vi "SpectrumAnn SCPI commands.vi"(11 "Path":path) -> (0 "error out":errorcluster, 2 "result string":string="3-19-2018", 3 "VISA Refnum out":refnum<visa-resource-name>)   [LabVIEW 2017]
uses:
  <vilib>/regexp/Match Regular Expression.xnode
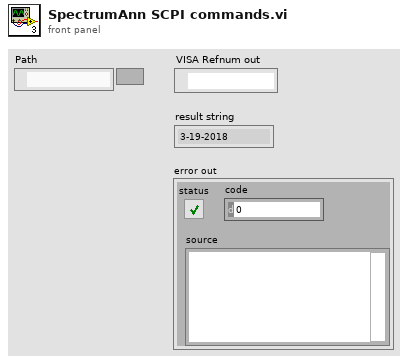
[diagram p1: front panel]
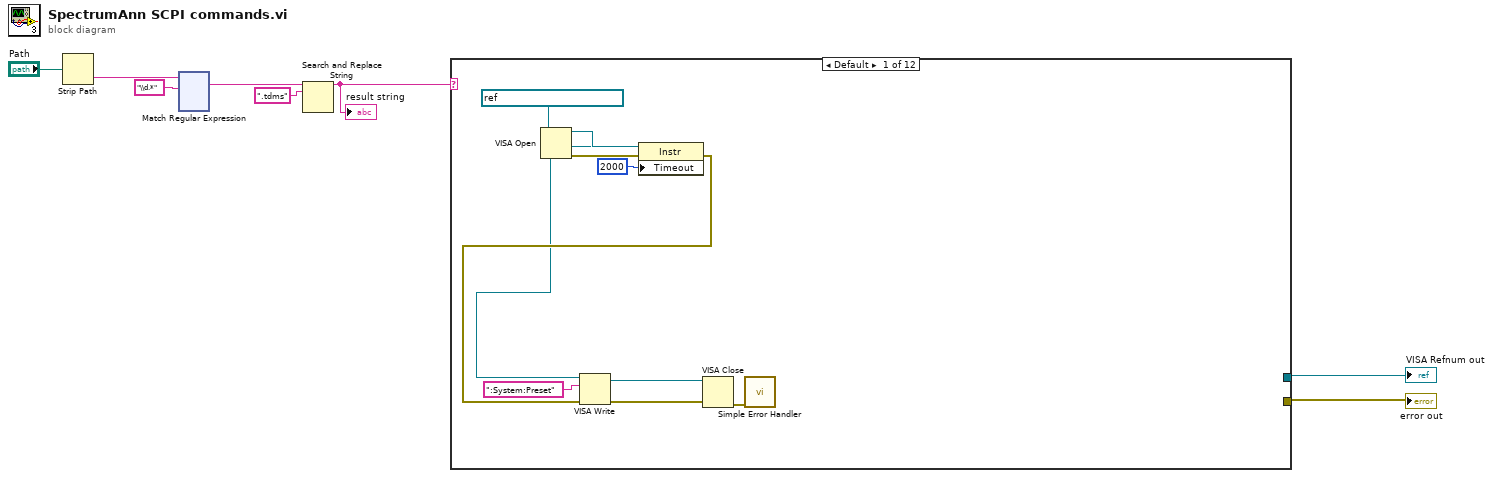
[diagram p0: block diagram]
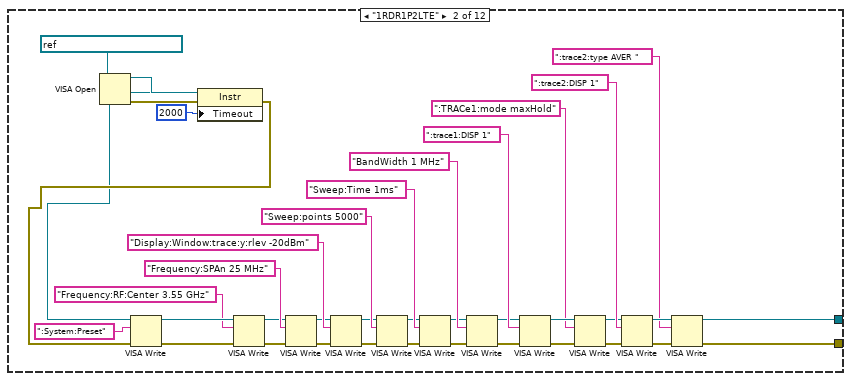
[diagram p2: hidden frame]
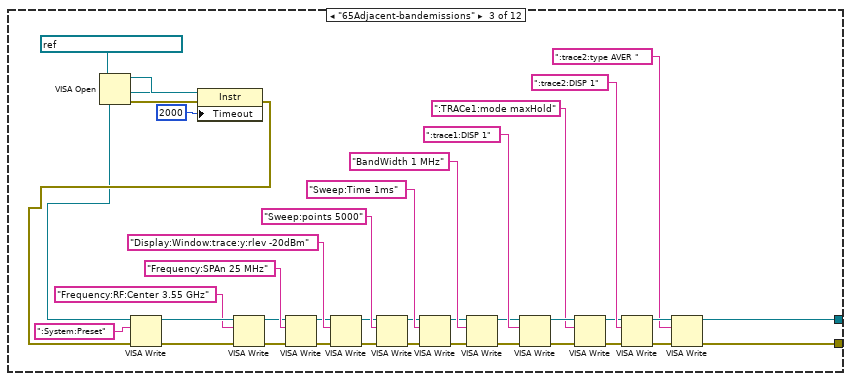
[diagram p3: hidden frame]
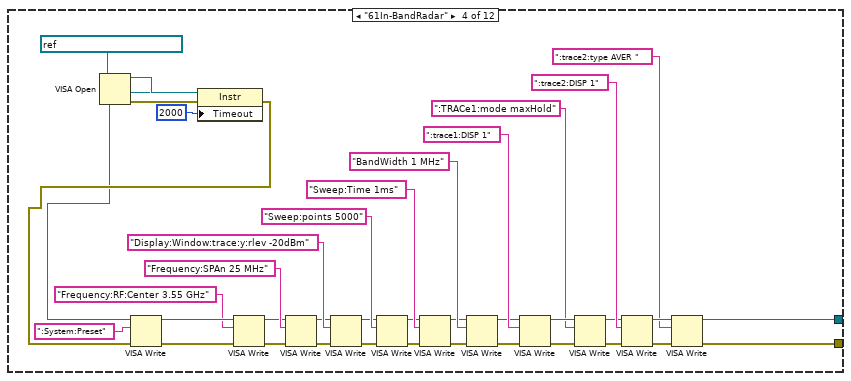
[diagram p4: hidden frame]
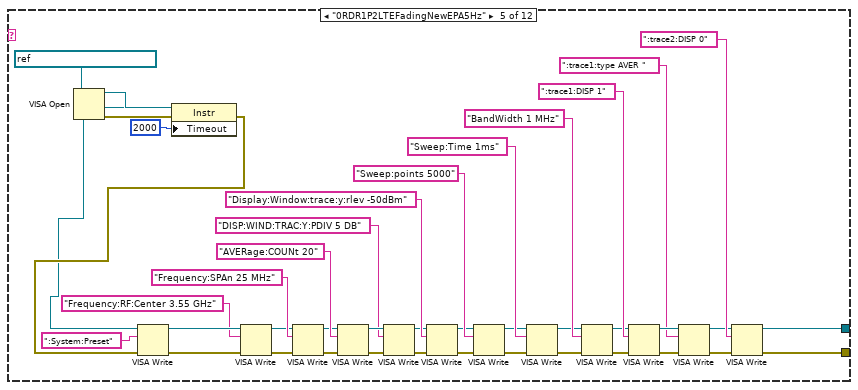
[diagram p5: hidden frame]
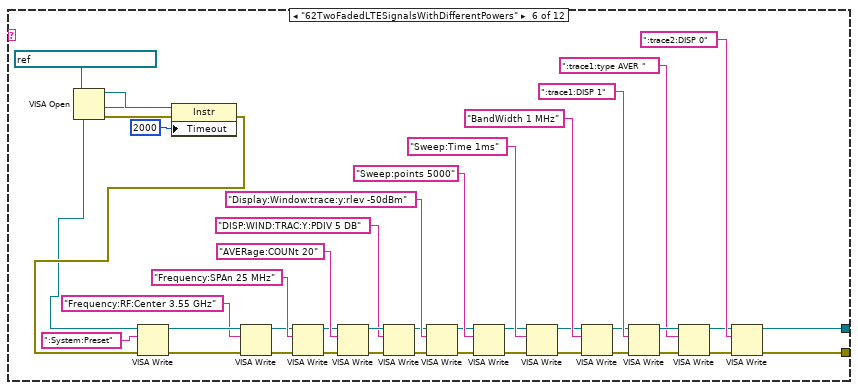
[diagram p6: hidden frame]
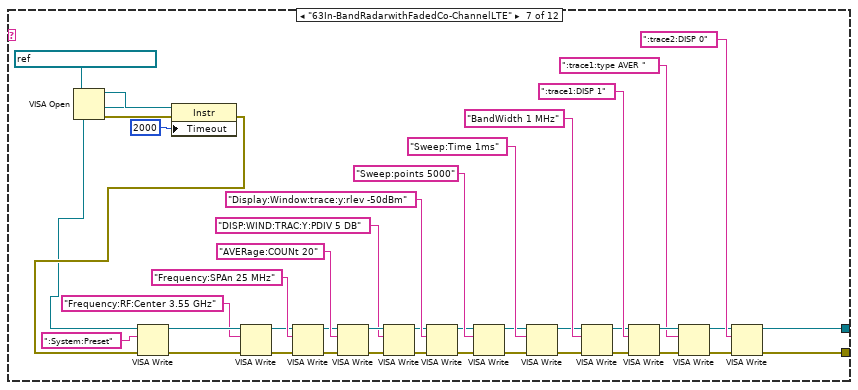
[diagram p7: hidden frame]
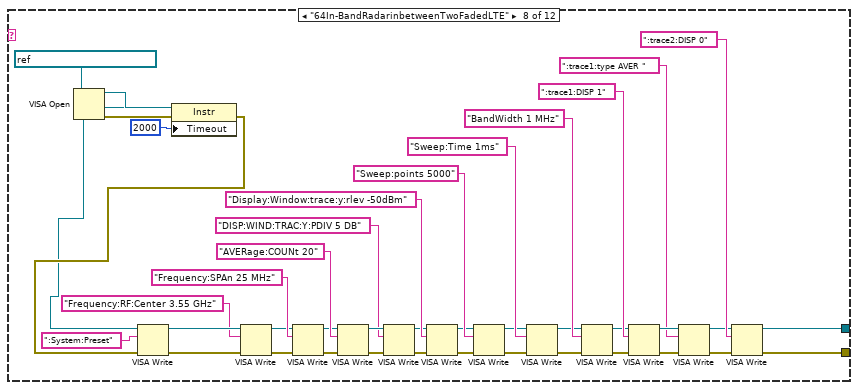
[diagram p8: hidden frame]
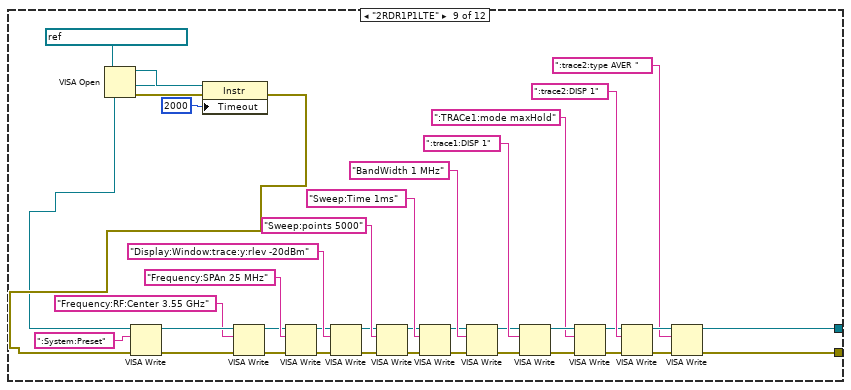
[diagram p9: hidden frame]
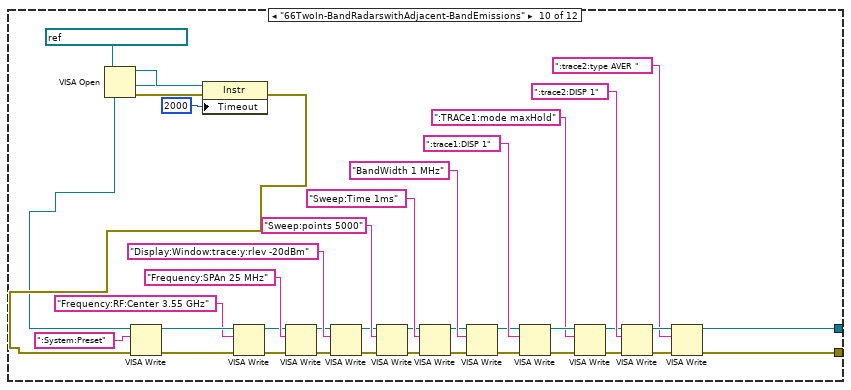
[diagram p10: hidden frame]
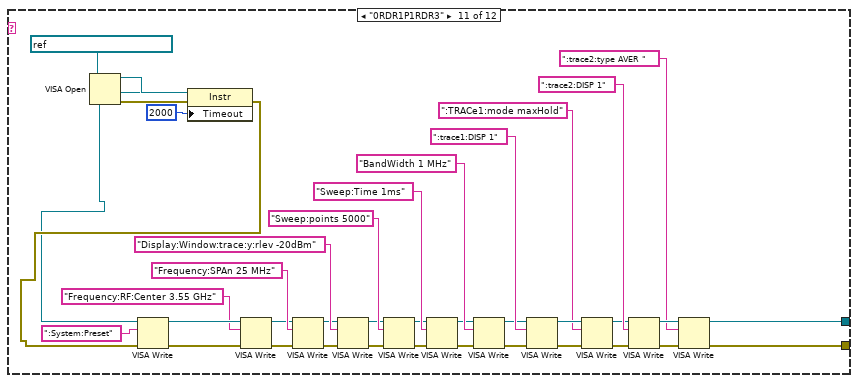
[diagram p11: hidden frame]
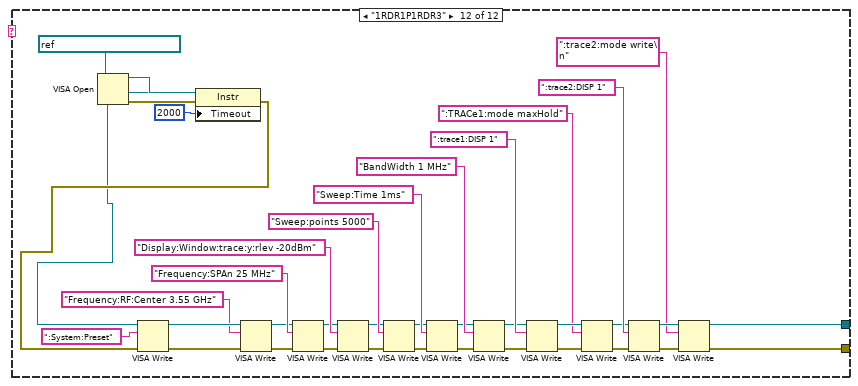
[diagram p12: hidden frame]
diagram:
  n1 = Strip Path(path="Path") -> (name=w5:string)  [unwired: 1 out]
  n2 = xnode "Match Regular Expression"("input string"=w5, "regular expression"="\\d.*") -> ("whole match"=w1:string)  [unwired: 4 in, 4 out]
  n3 = Search and Replace String(input string=w1, search string=".tdms") -> (result string=w6:string)  [unwired: 6 in, 3 out]
  "result string" <- w6
  n4 = case shown="Default" w6 {
    tunnel: [_ w25 w64 w103 w143 w185 w227 w269 w311 w350 w389 w428] -> w7
    tunnel: [_ w26 w65 w104 w142 w184 w226 w268 w310 w349 w388 w427] -> w8
    frame Default {
      n5 = VISA Open(VISA resource name=refnum<visa-resource-name> "SpecAnn-9010A-20100") -> (VISA resource name=w16:refnum<visa-resource-name>, error out=w15:errorcluster)  [unwired: 4 in]
      n6 = property class="Instr"(reference=w16, error in=w15, "Timeout"=u32 2000 ("General Settings:Timeout Value")) -> (reference out=w12:refnum<visa-resource-name>, error out=w13:errorcluster)
      n7 = VISA Write(VISA resource name=w12, write buffer=":System:Preset", error in (no error)=w13) -> (VISA resource name out=w10:refnum<visa-resource-name>, error out=w9:errorcluster)  [unwired: 1 out]
      n8 = VISA Close(VISA resource name=w10, error in (no error)=w9) -> (error out=w11:errorcluster)
      n9 = call <vilib>:"Simple Error Handler.vi"("error in (no error)"=w11) -> ()  [unwired: 4 in, 5 out]
    }
    frame "1RDR1P2LTE" {
      n10 = VISA Open(VISA resource name=refnum<visa-resource-name> "SpecAnn-9010A-20100") -> (VISA resource name=w23:refnum<visa-resource-name>, error out=w22:errorcluster)  [unwired: 4 in]
      n11 = property class="Instr"(reference=w23, error in=w22, "Timeout"=u32 2000 ("General Settings:Timeout Value")) -> (reference out=w19:refnum<visa-resource-name>, error out=w20:errorcluster)
      n12 = VISA Write(VISA resource name=w19, write buffer=":System:Preset", error in (no error)=w20) -> (VISA resource name out=w47:refnum<visa-resource-name>, error out=w46:errorcluster)  [unwired: 1 out]
      n13 = VISA Write(VISA resource name=w47, write buffer="Frequency:RF:Center 3.55 GHz", error in (no error)=w46) -> (VISA resource name out=w39:refnum<visa-resource-name>, error out=w30:errorcluster)  [unwired: 1 out]
      n14 = VISA Write(VISA resource name=w39, write buffer="Frequency:SPAn 25 MHz", error in (no error)=w30) -> (VISA resource name out=w38:refnum<visa-resource-name>, error out=w31:errorcluster)  [unwired: 1 out]
      n15 = VISA Write(VISA resource name=w38, write buffer="Display:Window:trace:y:rlev -20dBm", error in (no error)=w31) -> (VISA resource name out=w37:refnum<visa-resource-name>, error out=w32:errorcluster)  [unwired: 1 out]
      n16 = VISA Write(VISA resource name=w37, write buffer="Sweep:points 5000", error in (no error)=w32) -> (VISA resource name out=w36:refnum<visa-resource-name>, error out=w33:errorcluster)  [unwired: 1 out]
      n17 = VISA Write(VISA resource name=w36, write buffer="Sweep:Time 1ms", error in (no error)=w33) -> (VISA resource name out=w35:refnum<visa-resource-name>, error out=w34:errorcluster)  [unwired: 1 out]
      n18 = VISA Write(VISA resource name=w35, write buffer="BandWidth 1 MHz", error in (no error)=w34) -> (VISA resource name out=w28:refnum<visa-resource-name>, error out=w29:errorcluster)  [unwired: 1 out]
      n19 = VISA Write(VISA resource name=w28, write buffer=":trace1:DISP 1", error in (no error)=w29) -> (VISA resource name out=w53:refnum<visa-resource-name>, error out=w52:errorcluster)  [unwired: 1 out]
      n20 = VISA Write(VISA resource name=w53, write buffer=":TRACe1:mode maxHold", error in (no error)=w52) -> (VISA resource name out=w50:refnum<visa-resource-name>, error out=w49:errorcluster)  [unwired: 1 out]
      n21 = VISA Write(VISA resource name=w50, write buffer=":trace2:DISP 1", error in (no error)=w49) -> (VISA resource name out=w56:refnum<visa-resource-name>, error out=w57:errorcluster)  [unwired: 1 out]
      n22 = VISA Write(VISA resource name=w56, write buffer=":trace2:type AVER ", error in (no error)=w57) -> (VISA resource name out=w25:refnum<visa-resource-name>, error out=w26:errorcluster)  [unwired: 1 out]
    }
    frame "65Adjacent-bandemissions" {
      n23 = VISA Open(VISA resource name=refnum<visa-resource-name> "SpecAnn-9010A-20100") -> (VISA resource name=w62:refnum<visa-resource-name>, error out=w61:errorcluster)  [unwired: 4 in]
      n24 = property class="Instr"(reference=w62, error in=w61, "Timeout"=u32 2000 ("General Settings:Timeout Value")) -> (reference out=w58:refnum<visa-resource-name>, error out=w59:errorcluster)
      n25 = VISA Write(VISA resource name=w58, write buffer=":System:Preset", error in (no error)=w59) -> (VISA resource name out=w86:refnum<visa-resource-name>, error out=w85:errorcluster)  [unwired: 1 out]
      n26 = VISA Write(VISA resource name=w86, write buffer="Frequency:RF:Center 3.55 GHz", error in (no error)=w85) -> (VISA resource name out=w78:refnum<visa-resource-name>, error out=w69:errorcluster)  [unwired: 1 out]
      n27 = VISA Write(VISA resource name=w78, write buffer="Frequency:SPAn 25 MHz", error in (no error)=w69) -> (VISA resource name out=w77:refnum<visa-resource-name>, error out=w70:errorcluster)  [unwired: 1 out]
      n28 = VISA Write(VISA resource name=w77, write buffer="Display:Window:trace:y:rlev -20dBm", error in (no error)=w70) -> (VISA resource name out=w76:refnum<visa-resource-name>, error out=w71:errorcluster)  [unwired: 1 out]
      n29 = VISA Write(VISA resource name=w76, write buffer="Sweep:points 5000", error in (no error)=w71) -> (VISA resource name out=w75:refnum<visa-resource-name>, error out=w72:errorcluster)  [unwired: 1 out]
      n30 = VISA Write(VISA resource name=w75, write buffer="Sweep:Time 1ms", error in (no error)=w72) -> (VISA resource name out=w74:refnum<visa-resource-name>, error out=w73:errorcluster)  [unwired: 1 out]
      n31 = VISA Write(VISA resource name=w74, write buffer="BandWidth 1 MHz", error in (no error)=w73) -> (VISA resource name out=w67:refnum<visa-resource-name>, error out=w68:errorcluster)  [unwired: 1 out]
      n32 = VISA Write(VISA resource name=w67, write buffer=":trace1:DISP 1", error in (no error)=w68) -> (VISA resource name out=w92:refnum<visa-resource-name>, error out=w91:errorcluster)  [unwired: 1 out]
      n33 = VISA Write(VISA resource name=w92, write buffer=":TRACe1:mode maxHold", error in (no error)=w91) -> (VISA resource name out=w89:refnum<visa-resource-name>, error out=w88:errorcluster)  [unwired: 1 out]
      n34 = VISA Write(VISA resource name=w89, write buffer=":trace2:DISP 1", error in (no error)=w88) -> (VISA resource name out=w95:refnum<visa-resource-name>, error out=w96:errorcluster)  [unwired: 1 out]
      n35 = VISA Write(VISA resource name=w95, write buffer=":trace2:type AVER ", error in (no error)=w96) -> (VISA resource name out=w64:refnum<visa-resource-name>, error out=w65:errorcluster)  [unwired: 1 out]
    }
    frame "61In-BandRadar" {
      n36 = VISA Open(VISA resource name=refnum<visa-resource-name> "SpecAnn-9010A-20100") -> (VISA resource name=w101:refnum<visa-resource-name>, error out=w100:errorcluster)  [unwired: 4 in]
      n37 = property class="Instr"(reference=w101, error in=w100, "Timeout"=u32 2000 ("General Settings:Timeout Value")) -> (reference out=w97:refnum<visa-resource-name>, error out=w98:errorcluster)
      n38 = VISA Write(VISA resource name=w97, write buffer=":System:Preset", error in (no error)=w98) -> (VISA resource name out=w125:refnum<visa-resource-name>, error out=w124:errorcluster)  [unwired: 1 out]
      n39 = VISA Write(VISA resource name=w125, write buffer="Frequency:RF:Center 3.55 GHz", error in (no error)=w124) -> (VISA resource name out=w117:refnum<visa-resource-name>, error out=w108:errorcluster)  [unwired: 1 out]
      n40 = VISA Write(VISA resource name=w117, write buffer="Frequency:SPAn 25 MHz", error in (no error)=w108) -> (VISA resource name out=w116:refnum<visa-resource-name>, error out=w109:errorcluster)  [unwired: 1 out]
      n41 = VISA Write(VISA resource name=w116, write buffer="Display:Window:trace:y:rlev -20dBm", error in (no error)=w109) -> (VISA resource name out=w115:refnum<visa-resource-name>, error out=w110:errorcluster)  [unwired: 1 out]
      n42 = VISA Write(VISA resource name=w115, write buffer="Sweep:points 5000", error in (no error)=w110) -> (VISA resource name out=w114:refnum<visa-resource-name>, error out=w111:errorcluster)  [unwired: 1 out]
      n43 = VISA Write(VISA resource name=w114, write buffer="Sweep:Time 1ms", error in (no error)=w111) -> (VISA resource name out=w113:refnum<visa-resource-name>, error out=w112:errorcluster)  [unwired: 1 out]
      n44 = VISA Write(VISA resource name=w113, write buffer="BandWidth 1 MHz", error in (no error)=w112) -> (VISA resource name out=w106:refnum<visa-resource-name>, error out=w107:errorcluster)  [unwired: 1 out]
      n45 = VISA Write(VISA resource name=w106, write buffer=":trace1:DISP 1", error in (no error)=w107) -> (VISA resource name out=w131:refnum<visa-resource-name>, error out=w130:errorcluster)  [unwired: 1 out]
      n46 = VISA Write(VISA resource name=w131, write buffer=":TRACe1:mode maxHold", error in (no error)=w130) -> (VISA resource name out=w128:refnum<visa-resource-name>, error out=w127:errorcluster)  [unwired: 1 out]
      n47 = VISA Write(VISA resource name=w128, write buffer=":trace2:DISP 1", error in (no error)=w127) -> (VISA resource name out=w134:refnum<visa-resource-name>, error out=w135:errorcluster)  [unwired: 1 out]
      n48 = VISA Write(VISA resource name=w134, write buffer=":trace2:type AVER ", error in (no error)=w135) -> (VISA resource name out=w103:refnum<visa-resource-name>, error out=w104:errorcluster)  [unwired: 1 out]
    }
    frame "0RDR1P2LTEFadingNewEPA5Hz" {
      n49 = VISA Open(VISA resource name=refnum<visa-resource-name> "SpecAnn-9010A-20100") -> (VISA resource name=w140:refnum<visa-resource-name>, error out=w139:errorcluster)  [unwired: 4 in]
      n50 = property class="Instr"(reference=w140, error in=w139, "Timeout"=u32 2000 ("General Settings:Timeout Value")) -> (reference out=w136:refnum<visa-resource-name>, error out=w137:errorcluster)
      n51 = VISA Write(VISA resource name=w136, write buffer=":System:Preset", error in (no error)=w137) -> (VISA resource name out=w169:refnum<visa-resource-name>, error out=w168:errorcluster)  [unwired: 1 out]
      n52 = VISA Write(VISA resource name=w169, write buffer="Frequency:RF:Center 3.55 GHz", error in (no error)=w168) -> (VISA resource name out=w161:refnum<visa-resource-name>, error out=w154:errorcluster)  [unwired: 1 out]
      n53 = VISA Write(VISA resource name=w161, write buffer="Frequency:SPAn 25 MHz", error in (no error)=w154) -> (VISA resource name out=w150:refnum<visa-resource-name>, error out=w149:errorcluster)  [unwired: 1 out]
      n54 = VISA Write(VISA resource name=w150, write buffer="AVERage:COUNt 20", error in (no error)=w149) -> (VISA resource name out=w145:refnum<visa-resource-name>, error out=w146:errorcluster)  [unwired: 1 out]
      n55 = VISA Write(VISA resource name=w145, write buffer="DISP:WIND:TRAC:Y:PDIV 5 DB", error in (no error)=w146) -> (VISA resource name out=w148:refnum<visa-resource-name>, error out=w147:errorcluster)  [unwired: 1 out]
      n56 = VISA Write(VISA resource name=w148, write buffer="Display:Window:trace:y:rlev -50dBm", error in (no error)=w147) -> (VISA resource name out=w160:refnum<visa-resource-name>, error out=w155:errorcluster)  [unwired: 1 out]
      n57 = VISA Write(VISA resource name=w160, write buffer="Sweep:points 5000", error in (no error)=w155) -> (VISA resource name out=w159:refnum<visa-resource-name>, error out=w156:errorcluster)  [unwired: 1 out]
      n58 = VISA Write(VISA resource name=w159, write buffer="Sweep:Time 1ms", error in (no error)=w156) -> (VISA resource name out=w158:refnum<visa-resource-name>, error out=w157:errorcluster)  [unwired: 1 out]
      n59 = VISA Write(VISA resource name=w158, write buffer="BandWidth 1 MHz", error in (no error)=w157) -> (VISA resource name out=w152:refnum<visa-resource-name>, error out=w153:errorcluster)  [unwired: 1 out]
      n60 = VISA Write(VISA resource name=w152, write buffer=":trace1:DISP 1", error in (no error)=w153) -> (VISA resource name out=w175:refnum<visa-resource-name>, error out=w174:errorcluster)  [unwired: 1 out]
      n61 = VISA Write(VISA resource name=w175, write buffer=":trace1:type AVER ", error in (no error)=w174) -> (VISA resource name out=w172:refnum<visa-resource-name>, error out=w171:errorcluster)  [unwired: 1 out]
      n62 = VISA Write(VISA resource name=w172, write buffer=":trace2:DISP 0", error in (no error)=w171) -> (VISA resource name out=w143:refnum<visa-resource-name>, error out=w142:errorcluster)  [unwired: 1 out]
    }
    frame "62TwoFadedLTESignalsWithDifferentPowers" {
      n63 = VISA Open(VISA resource name=refnum<visa-resource-name> "SpecAnn-9010A-20100") -> (VISA resource name=w182:refnum<visa-resource-name>, error out=w181:errorcluster)  [unwired: 4 in]
      n64 = property class="Instr"(reference=w182, error in=w181, "Timeout"=u32 2000 ("General Settings:Timeout Value")) -> (reference out=w178:refnum<visa-resource-name>, error out=w179:errorcluster)
      n65 = VISA Write(VISA resource name=w178, write buffer=":System:Preset", error in (no error)=w179) -> (VISA resource name out=w211:refnum<visa-resource-name>, error out=w210:errorcluster)  [unwired: 1 out]
      n66 = VISA Write(VISA resource name=w211, write buffer="Frequency:RF:Center 3.55 GHz", error in (no error)=w210) -> (VISA resource name out=w203:refnum<visa-resource-name>, error out=w196:errorcluster)  [unwired: 1 out]
      n67 = VISA Write(VISA resource name=w203, write buffer="Frequency:SPAn 25 MHz", error in (no error)=w196) -> (VISA resource name out=w192:refnum<visa-resource-name>, error out=w191:errorcluster)  [unwired: 1 out]
      n68 = VISA Write(VISA resource name=w192, write buffer="AVERage:COUNt 20", error in (no error)=w191) -> (VISA resource name out=w187:refnum<visa-resource-name>, error out=w188:errorcluster)  [unwired: 1 out]
      n69 = VISA Write(VISA resource name=w187, write buffer="DISP:WIND:TRAC:Y:PDIV 5 DB", error in (no error)=w188) -> (VISA resource name out=w190:refnum<visa-resource-name>, error out=w189:errorcluster)  [unwired: 1 out]
      n70 = VISA Write(VISA resource name=w190, write buffer="Display:Window:trace:y:rlev -50dBm", error in (no error)=w189) -> (VISA resource name out=w202:refnum<visa-resource-name>, error out=w197:errorcluster)  [unwired: 1 out]
      n71 = VISA Write(VISA resource name=w202, write buffer="Sweep:points 5000", error in (no error)=w197) -> (VISA resource name out=w201:refnum<visa-resource-name>, error out=w198:errorcluster)  [unwired: 1 out]
      n72 = VISA Write(VISA resource name=w201, write buffer="Sweep:Time 1ms", error in (no error)=w198) -> (VISA resource name out=w200:refnum<visa-resource-name>, error out=w199:errorcluster)  [unwired: 1 out]
      n73 = VISA Write(VISA resource name=w200, write buffer="BandWidth 1 MHz", error in (no error)=w199) -> (VISA resource name out=w194:refnum<visa-resource-name>, error out=w195:errorcluster)  [unwired: 1 out]
      n74 = VISA Write(VISA resource name=w194, write buffer=":trace1:DISP 1", error in (no error)=w195) -> (VISA resource name out=w217:refnum<visa-resource-name>, error out=w216:errorcluster)  [unwired: 1 out]
      n75 = VISA Write(VISA resource name=w217, write buffer=":trace1:type AVER ", error in (no error)=w216) -> (VISA resource name out=w214:refnum<visa-resource-name>, error out=w213:errorcluster)  [unwired: 1 out]
      n76 = VISA Write(VISA resource name=w214, write buffer=":trace2:DISP 0", error in (no error)=w213) -> (VISA resource name out=w185:refnum<visa-resource-name>, error out=w184:errorcluster)  [unwired: 1 out]
    }
    frame "63In-BandRadarwithFadedCo-ChannelLTE" {
      n77 = VISA Open(VISA resource name=refnum<visa-resource-name> "SpecAnn-9010A-20100") -> (VISA resource name=w224:refnum<visa-resource-name>, error out=w223:errorcluster)  [unwired: 4 in]
      n78 = property class="Instr"(reference=w224, error in=w223, "Timeout"=u32 2000 ("General Settings:Timeout Value")) -> (reference out=w220:refnum<visa-resource-name>, error out=w221:errorcluster)
      n79 = VISA Write(VISA resource name=w220, write buffer=":System:Preset", error in (no error)=w221) -> (VISA resource name out=w253:refnum<visa-resource-name>, error out=w252:errorcluster)  [unwired: 1 out]
      n80 = VISA Write(VISA resource name=w253, write buffer="Frequency:RF:Center 3.55 GHz", error in (no error)=w252) -> (VISA resource name out=w245:refnum<visa-resource-name>, error out=w238:errorcluster)  [unwired: 1 out]
      n81 = VISA Write(VISA resource name=w245, write buffer="Frequency:SPAn 25 MHz", error in (no error)=w238) -> (VISA resource name out=w234:refnum<visa-resource-name>, error out=w233:errorcluster)  [unwired: 1 out]
      n82 = VISA Write(VISA resource name=w234, write buffer="AVERage:COUNt 20", error in (no error)=w233) -> (VISA resource name out=w229:refnum<visa-resource-name>, error out=w230:errorcluster)  [unwired: 1 out]
      n83 = VISA Write(VISA resource name=w229, write buffer="DISP:WIND:TRAC:Y:PDIV 5 DB", error in (no error)=w230) -> (VISA resource name out=w232:refnum<visa-resource-name>, error out=w231:errorcluster)  [unwired: 1 out]
      n84 = VISA Write(VISA resource name=w232, write buffer="Display:Window:trace:y:rlev -50dBm", error in (no error)=w231) -> (VISA resource name out=w244:refnum<visa-resource-name>, error out=w239:errorcluster)  [unwired: 1 out]
      n85 = VISA Write(VISA resource name=w244, write buffer="Sweep:points 5000", error in (no error)=w239) -> (VISA resource name out=w243:refnum<visa-resource-name>, error out=w240:errorcluster)  [unwired: 1 out]
      n86 = VISA Write(VISA resource name=w243, write buffer="Sweep:Time 1ms", error in (no error)=w240) -> (VISA resource name out=w242:refnum<visa-resource-name>, error out=w241:errorcluster)  [unwired: 1 out]
      n87 = VISA Write(VISA resource name=w242, write buffer="BandWidth 1 MHz", error in (no error)=w241) -> (VISA resource name out=w236:refnum<visa-resource-name>, error out=w237:errorcluster)  [unwired: 1 out]
      n88 = VISA Write(VISA resource name=w236, write buffer=":trace1:DISP 1", error in (no error)=w237) -> (VISA resource name out=w259:refnum<visa-resource-name>, error out=w258:errorcluster)  [unwired: 1 out]
      n89 = VISA Write(VISA resource name=w259, write buffer=":trace1:type AVER ", error in (no error)=w258) -> (VISA resource name out=w256:refnum<visa-resource-name>, error out=w255:errorcluster)  [unwired: 1 out]
      n90 = VISA Write(VISA resource name=w256, write buffer=":trace2:DISP 0", error in (no error)=w255) -> (VISA resource name out=w227:refnum<visa-resource-name>, error out=w226:errorcluster)  [unwired: 1 out]
    }
    frame "64In-BandRadarinbetweenTwoFadedLTE" {
      n91 = VISA Open(VISA resource name=refnum<visa-resource-name> "SpecAnn-9010A-20100") -> (VISA resource name=w266:refnum<visa-resource-name>, error out=w265:errorcluster)  [unwired: 4 in]
      n92 = property class="Instr"(reference=w266, error in=w265, "Timeout"=u32 2000 ("General Settings:Timeout Value")) -> (reference out=w262:refnum<visa-resource-name>, error out=w263:errorcluster)
      n93 = VISA Write(VISA resource name=w262, write buffer=":System:Preset", error in (no error)=w263) -> (VISA resource name out=w295:refnum<visa-resource-name>, error out=w294:errorcluster)  [unwired: 1 out]
      n94 = VISA Write(VISA resource name=w295, write buffer="Frequency:RF:Center 3.55 GHz", error in (no error)=w294) -> (VISA resource name out=w287:refnum<visa-resource-name>, error out=w280:errorcluster)  [unwired: 1 out]
      n95 = VISA Write(VISA resource name=w287, write buffer="Frequency:SPAn 25 MHz", error in (no error)=w280) -> (VISA resource name out=w276:refnum<visa-resource-name>, error out=w275:errorcluster)  [unwired: 1 out]
      n96 = VISA Write(VISA resource name=w276, write buffer="AVERage:COUNt 20", error in (no error)=w275) -> (VISA resource name out=w271:refnum<visa-resource-name>, error out=w272:errorcluster)  [unwired: 1 out]
      n97 = VISA Write(VISA resource name=w271, write buffer="DISP:WIND:TRAC:Y:PDIV 5 DB", error in (no error)=w272) -> (VISA resource name out=w274:refnum<visa-resource-name>, error out=w273:errorcluster)  [unwired: 1 out]
      n98 = VISA Write(VISA resource name=w274, write buffer="Display:Window:trace:y:rlev -50dBm", error in (no error)=w273) -> (VISA resource name out=w286:refnum<visa-resource-name>, error out=w281:errorcluster)  [unwired: 1 out]
      n99 = VISA Write(VISA resource name=w286, write buffer="Sweep:points 5000", error in (no error)=w281) -> (VISA resource name out=w285:refnum<visa-resource-name>, error out=w282:errorcluster)  [unwired: 1 out]
      n100 = VISA Write(VISA resource name=w285, write buffer="Sweep:Time 1ms", error in (no error)=w282) -> (VISA resource name out=w284:refnum<visa-resource-name>, error out=w283:errorcluster)  [unwired: 1 out]
      n101 = VISA Write(VISA resource name=w284, write buffer="BandWidth 1 MHz", error in (no error)=w283) -> (VISA resource name out=w278:refnum<visa-resource-name>, error out=w279:errorcluster)  [unwired: 1 out]
      n102 = VISA Write(VISA resource name=w278, write buffer=":trace1:DISP 1", error in (no error)=w279) -> (VISA resource name out=w301:refnum<visa-resource-name>, error out=w300:errorcluster)  [unwired: 1 out]
      n103 = VISA Write(VISA resource name=w301, write buffer=":trace1:type AVER ", error in (no error)=w300) -> (VISA resource name out=w298:refnum<visa-resource-name>, error out=w297:errorcluster)  [unwired: 1 out]
      n104 = VISA Write(VISA resource name=w298, write buffer=":trace2:DISP 0", error in (no error)=w297) -> (VISA resource name out=w269:refnum<visa-resource-name>, error out=w268:errorcluster)  [unwired: 1 out]
    }
    frame "2RDR1P1LTE" {
      n105 = VISA Open(VISA resource name=refnum<visa-resource-name> "SpecAnn-9010A-20100") -> (VISA resource name=w308:refnum<visa-resource-name>, error out=w307:errorcluster)  [unwired: 4 in]
      n106 = property class="Instr"(reference=w308, error in=w307, "Timeout"=u32 2000 ("General Settings:Timeout Value")) -> (reference out=w304:refnum<visa-resource-name>, error out=w305:errorcluster)
      n107 = VISA Write(VISA resource name=w304, write buffer=":System:Preset", error in (no error)=w305) -> (VISA resource name out=w332:refnum<visa-resource-name>, error out=w331:errorcluster)  [unwired: 1 out]
      n108 = VISA Write(VISA resource name=w332, write buffer="Frequency:RF:Center 3.55 GHz", error in (no error)=w331) -> (VISA resource name out=w324:refnum<visa-resource-name>, error out=w315:errorcluster)  [unwired: 1 out]
      n109 = VISA Write(VISA resource name=w324, write buffer="Frequency:SPAn 25 MHz", error in (no error)=w315) -> (VISA resource name out=w323:refnum<visa-resource-name>, error out=w316:errorcluster)  [unwired: 1 out]
      n110 = VISA Write(VISA resource name=w323, write buffer="Display:Window:trace:y:rlev -20dBm", error in (no error)=w316) -> (VISA resource name out=w322:refnum<visa-resource-name>, error out=w317:errorcluster)  [unwired: 1 out]
      n111 = VISA Write(VISA resource name=w322, write buffer="Sweep:points 5000", error in (no error)=w317) -> (VISA resource name out=w321:refnum<visa-resource-name>, error out=w318:errorcluster)  [unwired: 1 out]
      n112 = VISA Write(VISA resource name=w321, write buffer="Sweep:Time 1ms", error in (no error)=w318) -> (VISA resource name out=w320:refnum<visa-resource-name>, error out=w319:errorcluster)  [unwired: 1 out]
      n113 = VISA Write(VISA resource name=w320, write buffer="BandWidth 1 MHz", error in (no error)=w319) -> (VISA resource name out=w313:refnum<visa-resource-name>, error out=w314:errorcluster)  [unwired: 1 out]
      n114 = VISA Write(VISA resource name=w313, write buffer=":trace1:DISP 1", error in (no error)=w314) -> (VISA resource name out=w338:refnum<visa-resource-name>, error out=w337:errorcluster)  [unwired: 1 out]
      n115 = VISA Write(VISA resource name=w338, write buffer=":TRACe1:mode maxHold", error in (no error)=w337) -> (VISA resource name out=w335:refnum<visa-resource-name>, error out=w334:errorcluster)  [unwired: 1 out]
      n116 = VISA Write(VISA resource name=w335, write buffer=":trace2:DISP 1", error in (no error)=w334) -> (VISA resource name out=w341:refnum<visa-resource-name>, error out=w342:errorcluster)  [unwired: 1 out]
      n117 = VISA Write(VISA resource name=w341, write buffer=":trace2:type AVER ", error in (no error)=w342) -> (VISA resource name out=w311:refnum<visa-resource-name>, error out=w310:errorcluster)  [unwired: 1 out]
    }
    frame "66TwoIn-BandRadarswithAdjacent-BandEmissions" {
      n118 = VISA Open(VISA resource name=refnum<visa-resource-name> "SpecAnn-9010A-20100") -> (VISA resource name=w347:refnum<visa-resource-name>, error out=w346:errorcluster)  [unwired: 4 in]
      n119 = property class="Instr"(reference=w347, error in=w346, "Timeout"=u32 2000 ("General Settings:Timeout Value")) -> (reference out=w343:refnum<visa-resource-name>, error out=w344:errorcluster)
      n120 = VISA Write(VISA resource name=w343, write buffer=":System:Preset", error in (no error)=w344) -> (VISA resource name out=w371:refnum<visa-resource-name>, error out=w370:errorcluster)  [unwired: 1 out]
      n121 = VISA Write(VISA resource name=w371, write buffer="Frequency:RF:Center 3.55 GHz", error in (no error)=w370) -> (VISA resource name out=w363:refnum<visa-resource-name>, error out=w354:errorcluster)  [unwired: 1 out]
      n122 = VISA Write(VISA resource name=w363, write buffer="Frequency:SPAn 25 MHz", error in (no error)=w354) -> (VISA resource name out=w362:refnum<visa-resource-name>, error out=w355:errorcluster)  [unwired: 1 out]
      n123 = VISA Write(VISA resource name=w362, write buffer="Display:Window:trace:y:rlev -20dBm", error in (no error)=w355) -> (VISA resource name out=w361:refnum<visa-resource-name>, error out=w356:errorcluster)  [unwired: 1 out]
      n124 = VISA Write(VISA resource name=w361, write buffer="Sweep:points 5000", error in (no error)=w356) -> (VISA resource name out=w360:refnum<visa-resource-name>, error out=w357:errorcluster)  [unwired: 1 out]
      n125 = VISA Write(VISA resource name=w360, write buffer="Sweep:Time 1ms", error in (no error)=w357) -> (VISA resource name out=w359:refnum<visa-resource-name>, error out=w358:errorcluster)  [unwired: 1 out]
      n126 = VISA Write(VISA resource name=w359, write buffer="BandWidth 1 MHz", error in (no error)=w358) -> (VISA resource name out=w352:refnum<visa-resource-name>, error out=w353:errorcluster)  [unwired: 1 out]
      n127 = VISA Write(VISA resource name=w352, write buffer=":trace1:DISP 1", error in (no error)=w353) -> (VISA resource name out=w377:refnum<visa-resource-name>, error out=w376:errorcluster)  [unwired: 1 out]
      n128 = VISA Write(VISA resource name=w377, write buffer=":TRACe1:mode maxHold", error in (no error)=w376) -> (VISA resource name out=w374:refnum<visa-resource-name>, error out=w373:errorcluster)  [unwired: 1 out]
      n129 = VISA Write(VISA resource name=w374, write buffer=":trace2:DISP 1", error in (no error)=w373) -> (VISA resource name out=w380:refnum<visa-resource-name>, error out=w381:errorcluster)  [unwired: 1 out]
      n130 = VISA Write(VISA resource name=w380, write buffer=":trace2:type AVER ", error in (no error)=w381) -> (VISA resource name out=w350:refnum<visa-resource-name>, error out=w349:errorcluster)  [unwired: 1 out]
    }
    frame "0RDR1P1RDR3" {
      n131 = VISA Open(VISA resource name=refnum<visa-resource-name> "SpecAnn-9010A-20100") -> (VISA resource name=w386:refnum<visa-resource-name>, error out=w385:errorcluster)  [unwired: 4 in]
      n132 = property class="Instr"(reference=w386, error in=w385, "Timeout"=u32 2000 ("General Settings:Timeout Value")) -> (reference out=w382:refnum<visa-resource-name>, error out=w383:errorcluster)
      n133 = VISA Write(VISA resource name=w382, write buffer=":System:Preset", error in (no error)=w383) -> (VISA resource name out=w410:refnum<visa-resource-name>, error out=w409:errorcluster)  [unwired: 1 out]
      n134 = VISA Write(VISA resource name=w410, write buffer="Frequency:RF:Center 3.55 GHz", error in (no error)=w409) -> (VISA resource name out=w402:refnum<visa-resource-name>, error out=w393:errorcluster)  [unwired: 1 out]
      n135 = VISA Write(VISA resource name=w402, write buffer="Frequency:SPAn 25 MHz", error in (no error)=w393) -> (VISA resource name out=w401:refnum<visa-resource-name>, error out=w394:errorcluster)  [unwired: 1 out]
      n136 = VISA Write(VISA resource name=w401, write buffer="Display:Window:trace:y:rlev -20dBm", error in (no error)=w394) -> (VISA resource name out=w400:refnum<visa-resource-name>, error out=w395:errorcluster)  [unwired: 1 out]
      n137 = VISA Write(VISA resource name=w400, write buffer="Sweep:points 5000", error in (no error)=w395) -> (VISA resource name out=w399:refnum<visa-resource-name>, error out=w396:errorcluster)  [unwired: 1 out]
      n138 = VISA Write(VISA resource name=w399, write buffer="Sweep:Time 1ms", error in (no error)=w396) -> (VISA resource name out=w398:refnum<visa-resource-name>, error out=w397:errorcluster)  [unwired: 1 out]
      n139 = VISA Write(VISA resource name=w398, write buffer="BandWidth 1 MHz", error in (no error)=w397) -> (VISA resource name out=w391:refnum<visa-resource-name>, error out=w392:errorcluster)  [unwired: 1 out]
      n140 = VISA Write(VISA resource name=w391, write buffer=":trace1:DISP 1", error in (no error)=w392) -> (VISA resource name out=w416:refnum<visa-resource-name>, error out=w415:errorcluster)  [unwired: 1 out]
      n141 = VISA Write(VISA resource name=w416, write buffer=":TRACe1:mode maxHold", error in (no error)=w415) -> (VISA resource name out=w413:refnum<visa-resource-name>, error out=w412:errorcluster)  [unwired: 1 out]
      n142 = VISA Write(VISA resource name=w413, write buffer=":trace2:DISP 1", error in (no error)=w412) -> (VISA resource name out=w419:refnum<visa-resource-name>, error out=w420:errorcluster)  [unwired: 1 out]
      n143 = VISA Write(VISA resource name=w419, write buffer=":trace2:type AVER ", error in (no error)=w420) -> (VISA resource name out=w389:refnum<visa-resource-name>, error out=w388:errorcluster)  [unwired: 1 out]
    }
    frame "1RDR1P1RDR3" {
      n144 = VISA Open(VISA resource name=refnum<visa-resource-name> "SpecAnn-9010A-20100") -> (VISA resource name=w425:refnum<visa-resource-name>, error out=w424:errorcluster)  [unwired: 4 in]
      n145 = property class="Instr"(reference=w425, error in=w424, "Timeout"=u32 2000 ("General Settings:Timeout Value")) -> (reference out=w421:refnum<visa-resource-name>, error out=w422:errorcluster)
      n146 = VISA Write(VISA resource name=w421, write buffer=":System:Preset", error in (no error)=w422) -> (VISA resource name out=w449:refnum<visa-resource-name>, error out=w448:errorcluster)  [unwired: 1 out]
      n147 = VISA Write(VISA resource name=w449, write buffer="Frequency:RF:Center 3.55 GHz", error in (no error)=w448) -> (VISA resource name out=w441:refnum<visa-resource-name>, error out=w432:errorcluster)  [unwired: 1 out]
      n148 = VISA Write(VISA resource name=w441, write buffer="Frequency:SPAn 25 MHz", error in (no error)=w432) -> (VISA resource name out=w440:refnum<visa-resource-name>, error out=w433:errorcluster)  [unwired: 1 out]
      n149 = VISA Write(VISA resource name=w440, write buffer="Display:Window:trace:y:rlev -20dBm", error in (no error)=w433) -> (VISA resource name out=w439:refnum<visa-resource-name>, error out=w434:errorcluster)  [unwired: 1 out]
      n150 = VISA Write(VISA resource name=w439, write buffer="Sweep:points 5000", error in (no error)=w434) -> (VISA resource name out=w438:refnum<visa-resource-name>, error out=w435:errorcluster)  [unwired: 1 out]
      n151 = VISA Write(VISA resource name=w438, write buffer="Sweep:Time 1ms", error in (no error)=w435) -> (VISA resource name out=w437:refnum<visa-resource-name>, error out=w436:errorcluster)  [unwired: 1 out]
      n152 = VISA Write(VISA resource name=w437, write buffer="BandWidth 1 MHz", error in (no error)=w436) -> (VISA resource name out=w430:refnum<visa-resource-name>, error out=w431:errorcluster)  [unwired: 1 out]
      n153 = VISA Write(VISA resource name=w430, write buffer=":trace1:DISP 1", error in (no error)=w431) -> (VISA resource name out=w455:refnum<visa-resource-name>, error out=w454:errorcluster)  [unwired: 1 out]
      n154 = VISA Write(VISA resource name=w455, write buffer=":TRACe1:mode maxHold", error in (no error)=w454) -> (VISA resource name out=w452:refnum<visa-resource-name>, error out=w451:errorcluster)  [unwired: 1 out]
      n155 = VISA Write(VISA resource name=w452, write buffer=":trace2:DISP 1", error in (no error)=w451) -> (VISA resource name out=w458:refnum<visa-resource-name>, error out=w459:errorcluster)  [unwired: 1 out]
      n156 = VISA Write(VISA resource name=w458, write buffer=":trace2:mode write\n", error in (no error)=w459) -> (VISA resource name out=w428:refnum<visa-resource-name>, error out=w427:errorcluster)  [unwired: 1 out]
    }
  }
  "error out" <- w8
  "VISA Refnum out" <- w7
